vi "Increment head position.vi"(9 "Direction":string, 11 "H in":i32[](array[numeric])) -> (3 "H out":i32[](array[numeric]))   [LabVIEW 2020]
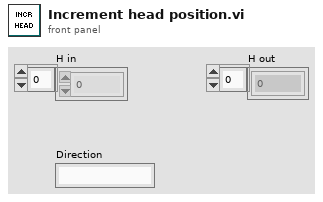
[diagram p1: front panel]
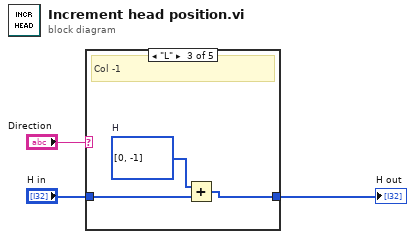
[diagram p0: block diagram]
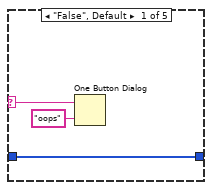
[diagram p2: hidden frame]
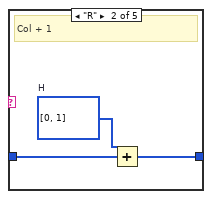
[diagram p3: hidden frame]
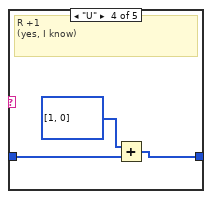
[diagram p4: hidden frame]
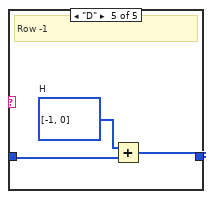
[diagram p5: hidden frame]
diagram:
  n1 = case shown="\"L\"" "Direction" {
    selector: "Direction" -> [w5 _ _ _ _]
    tunnel: "H in" -> [w6 w8 w12 w14 w17]
    tunnel: [w6 w7 w10 w13 w16] -> w3
    frame "False", Default {
      n2 = One Button Dialog(message=w5, button name ("OK")="oops") -> ()  [unwired: 1 out]
    }
    frame "R" {
      w9 = i32[] [0, 1]  # H
      # "Col + 1"
      n3 = Add(x=w9, y=w8) -> (x+y=w7:i32[])
    }
    frame "L" {
      w11 = i32[] [0, -1]  # H
      # "Col -1"
      n4 = Add(x=w11, y=w12) -> (x+y=w10:i32[])
    }
    frame "U" {
      # "R +1\n(yes, I know)"
      n5 = Add(x=i32[] [1, 0] ("H"), y=w14) -> (x+y=w13:i32[])
    }
    frame "D" {
      w18 = i32[] [-1, 0]  # H
      # "Row -1"
      n6 = Add(x=w18, y=w17) -> (x+y=w16:i32[])
    }
  }
  "H out" <- w3
